vi "40-295-121-10_16.vi"(7 "Resistance Value":u32[](array[numeric])=[1000, 2000, 3000, 4000, 5000, 6000, 7000, 8000, 9000, 10000], 8 "error in (no error)":errorcluster, 11 "VISA resource name":refnum<visa-resource-name>="PXI25::11::INSTR") -> (0 "error out":errorcluster={"status"=FALSE, "code"=0, "source"="pipx40 Close.vi"})   [LabVIEW 2011]
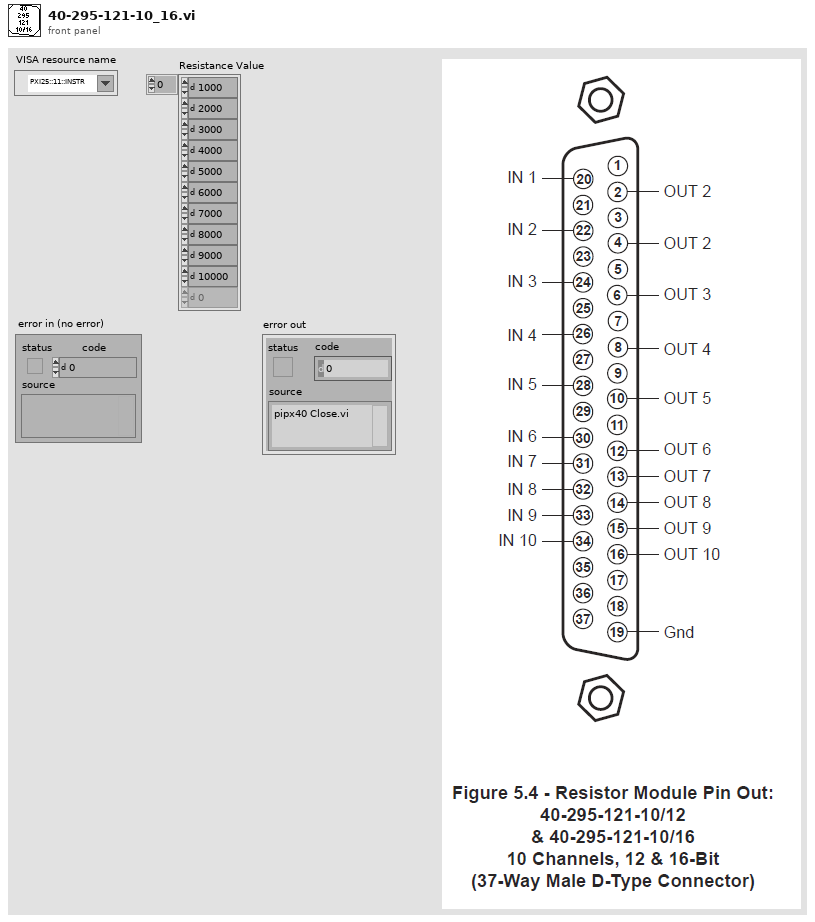
[diagram p1: front panel]
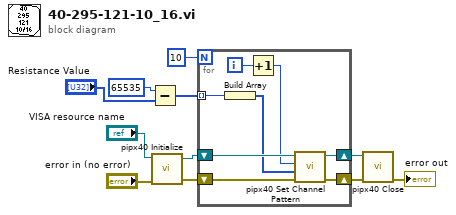
[diagram p0: block diagram]
diagram:
  n1 = Subtract(x=u32 65535 ("y"), y="Resistance Value") -> (x-y=w2:u32[])
  n2 = call "pipx40 Initialize.vi"("error in (no error)"="error in (no error)", "resource name"="VISA resource name") -> ("error out"=w5:errorcluster, "instrument handle out"=w6:refnum<visa-resource-name>)  [unwired: 2 in, 1 out]
  n3 = for {
    N: u32 10 ("output subunits") -> [_]
    shift-right: [w15] -> w10
    shift-left: w5 -> [w17]
    shift-right: [w14] -> w11
    shift-left: w6 -> [w18]
    tunnel: w2 -> [w12] mode=indexing
    i -> [w19]
    n4 = Build Array(w12) -> (w13:u32[])
    n5 = Increment(x=w19) -> (x+1=w16:i32)
    n6 = call "pipx40 Set Channel Pattern.vi"("error in (no error)"=w17, "pattern"=w13, "subunit number"=w16, "instrument handle"=w18) -> ("error out"=w15:errorcluster, "instrument handle out"=w14:refnum<visa-resource-name>)  [unwired: 1 in, 1 out]
  }
  n7 = call "pipx40 Close.vi"("error in (no error)"=w10, "instrument handle"=w11) -> ("error out"=→"error out":errorcluster)  [unwired: 8 in, 1 out]
